vi "async metadata make.vi"(8 "error in (no error)":errorcluster, 11 "handle":u64) -> (0 "error out":errorcluster, 2 "function return":u32(ring), 3 "handle out":u64)   [LabVIEW 2023, in "uhd.lvlib"]
doc: "UHD_API uhd_error uhd_async_metadata_make(uhd_async_metadata_handle* handle);"
uses:
  <userlib>/uhd/uhd.lvlib
  <userlib>/uhd/uhd.dll
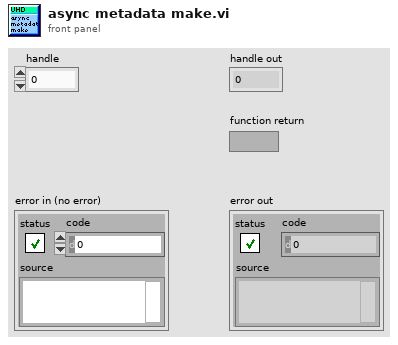
[diagram p1: front panel]
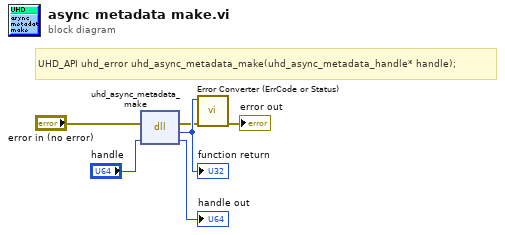
[diagram p0: block diagram]
diagram:
  # "UHD_API uhd_error uhd_async_metadata_make(uhd_async_metadata_handle* handle);"
  n1 = dll-call lib="C:/Program Files/National Instruments/LabVIEW 2023/user.lib/uhd/uhd.*" fn="uhd_async_metadata_make"(error in="error in (no error)", "handle"="handle") -> (error out=w2:errorcluster, w6:u32, "handle"=→"handle out":u64)  [unwired: 2 in, 1 out]
  "function return" <- w6
  n2 = call <userlib>:"Error Converter (ErrCode or Status).vi"("error in (no error)"=w2, "error code"=w6) -> ("error out"=→"error out":errorcluster)  [unwired: 9 in]
